vi "GenerateFilenames_2P.vi"(7 "path":path) -> (0 "WebCam Path":path, 1 "Whisker Path":path, 2 "TDMS Path":path, 3 "MScan Path":path, 5 "Analog file name":string="F:\\Data\\130725_14_35_2625", 6 "Pupil Path":path)   [LabVIEW 2020]
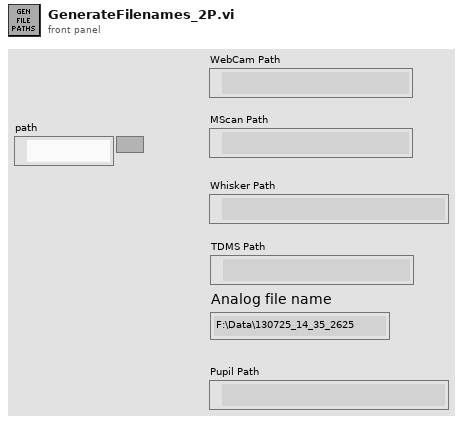
[diagram p1: front panel]
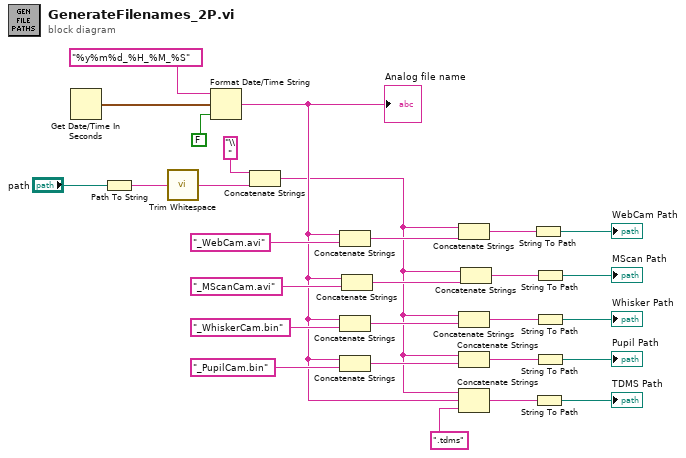
[diagram p0: block diagram]
diagram:
  n1 = Get Date/Time In Seconds() -> (seconds since 1Jan1904=w27:timestamp)
  n2 = Path To String(path="path") -> (string=w15:string)
  n3 = call <vilib>:"Trim Whitespace.vi"("string"=w15) -> ("trimmed string"=w13:string)  [unwired: 1 in]
  n4 = Format Date/Time String(time format string (%c)="%y%m%d_%H_%M_%S", seconds (now)=w27, UTC format=FALSE) -> (date/time string=w3:string)
  "Analog file name" <- w3
  n5 = Concatenate Strings(w13, "\\" ("string")) -> (w2:string)
  n6 = Concatenate Strings(w3, "_WebCam.avi") -> (w25:string)
  n7 = Concatenate Strings(w3, "_WhiskerCam.bin" ("string")) -> (w22:string)
  n8 = Concatenate Strings(w3, "_PupilCam.bin" ("string")) -> (w5:string)
  n9 = Concatenate Strings(w3, "_MScanCam.avi") -> (w10:string)
  n10 = Concatenate Strings(w2, w25) -> (w24:string)
  n11 = Concatenate Strings(w2, w22) -> (w21:string)
  n12 = Concatenate Strings(w2, w5) -> (w4:string)
  n13 = Concatenate Strings(w2, w3, ".tdms" ("string")) -> (w16:string)
  n14 = Concatenate Strings(w2, w10) -> (w9:string)
  n15 = String To Path(string=w24) -> (path=→"WebCam Path":path)
  n16 = String To Path(string=w16) -> (path=→"TDMS Path":path)
  n17 = String To Path(string=w9) -> (path=→"MScan Path":path)
  n18 = String To Path(string=w21) -> (path=→"Whisker Path":path)
  n19 = String To Path(string=w4) -> (path=→"Pupil Path":path)
